vi "Microsteps to Degrees (SubVI).vi"(4 "Microsteps":dbl) -> (1 "Numeric":dbl)   [LabVIEW 2012]
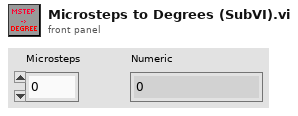
[diagram p1: front panel]
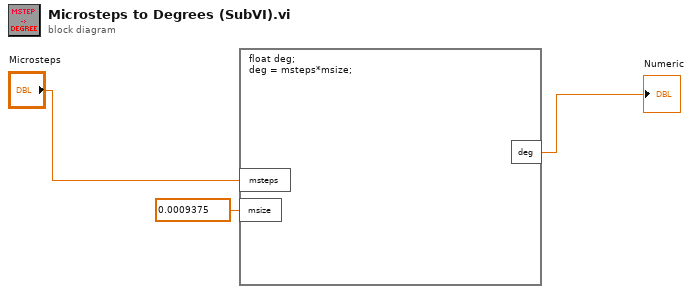
[diagram p0: block diagram]
diagram:
  n1 = formula code="float deg;\ndeg = msteps*msize;"("msteps"="Microsteps", "msize"=0.0009375 ("input variable")) -> ("deg"=→"Numeric":dbl)
